vi "decision.vi"(8 "offset":fxp<+/-,64,32>, 10 "weights":fxp<+/-,64,32>[](array[numeric]), 11 "inputs":fxp<+/-,64,32>[](array[numeric])) -> (2 "decision":fxp<+/-,64,32>)   [LabVIEW 2014]
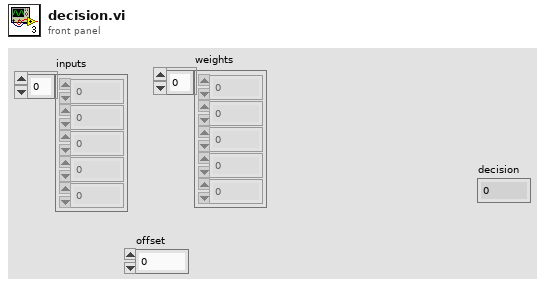
[diagram p1: front panel]
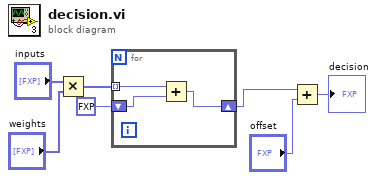
[diagram p0: block diagram]
diagram:
  n1 = Multiply(x="inputs", y="weights") -> (x*y=w3:fxp<+/-,64,32>[])
  n2 = for {
    tunnel: w3 -> [w10] mode=indexing
    shift-right: [w8] -> w1
    shift-left: fxp<+/-,64,32> 0.0 -> [w9]
    n3 = Add(x=w10, y=w9) -> (x+y=w8:fxp<+/-,64,32>)
  }
  n4 = Add(x=w1, y="offset") -> (x+y=→"decision":fxp<+/-,64,32>)
